vi "automationopen.vi"   [LabVIEW 2014]
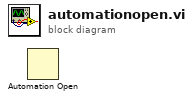
[diagram p0: block diagram]
diagram:
  n1 = Automation Open() -> ()  [unwired: 4 in, 2 out]
